vi "fg_stop.vi"(8 "error in (no error)":errorcluster) -> (0 "error out":errorcluster, 3 "stop_event":refnum<user-event>)   [LabVIEW 2015, in "example_01.lvlib"]
uses:
  example_01.lvlib
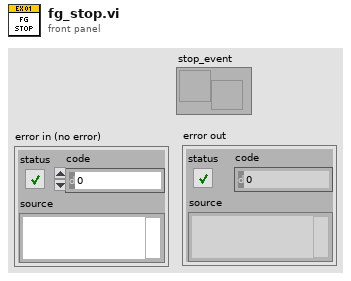
[diagram p1: front panel]
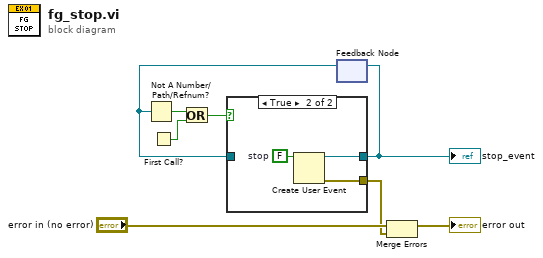
[diagram p0: block diagram]
diagram:
  n1 = First Call?() -> (First Call?: T/F=w8:bool)
  n2 = feedback #1() -> (w4:refnum<user-event>)  [unwired: 1 in]
  n3 = Not A Number/Path/Refnum?(number/path/refnum=w4) -> (NaN/Path/Refnum?=w7:bool)
  n4 = Or(x=w7, y=w8) -> (x .or. y?=w5:bool)
  n5 = case shown="True" w5 {
    tunnel: [w9 w11] -> w6
    tunnel: w4 -> [w9 _]
    tunnel: [_ w10] -> w1
    frame False {
    }
    frame True {
      w12 = FALSE  # stop
      n6 = Create User Event(user event datatype=w12) -> (user event=w11:refnum<user-event>, error out=w10:errorcluster)  [unwired: 1 in]
    }
  }
  "stop_event" <- w6
  n7 = feedback-in #1(w6) -> ()
  n8 = Merge Errors("error in (no error)", w1) -> (→"error out":errorcluster)
